vi "3D Point Cloud.vi"(0 "3D Information Cluster (X,Y,Z)":cluster{dbl[], dbl[], dbl[]}) -> ()   [LabVIEW 2010, in "Kinect_API.lvlib"]
doc: "This VI shows how to use the 3D Scatter Plot."
uses:
  Kinect_API.lvlib
  <vilib>/Math Plots/3D Math Plots/3D Scatter/3D Scatter XCtrl/3D Scatter.xctl
  <vilib>/Math Plots/3D Math Plots/3D Scatter/3D Scatter Datatype/Public/Plot Helper (Vector).vi
  <vilib>/Math Plots/3D Math Plots/3D Scatter/3D Scatter Datatype/3D Scatter Datatype.lvclass
panel:
  out "3D Scatter":refnum<class "3D Plot Datatype.lvclass">[](xcontrol)
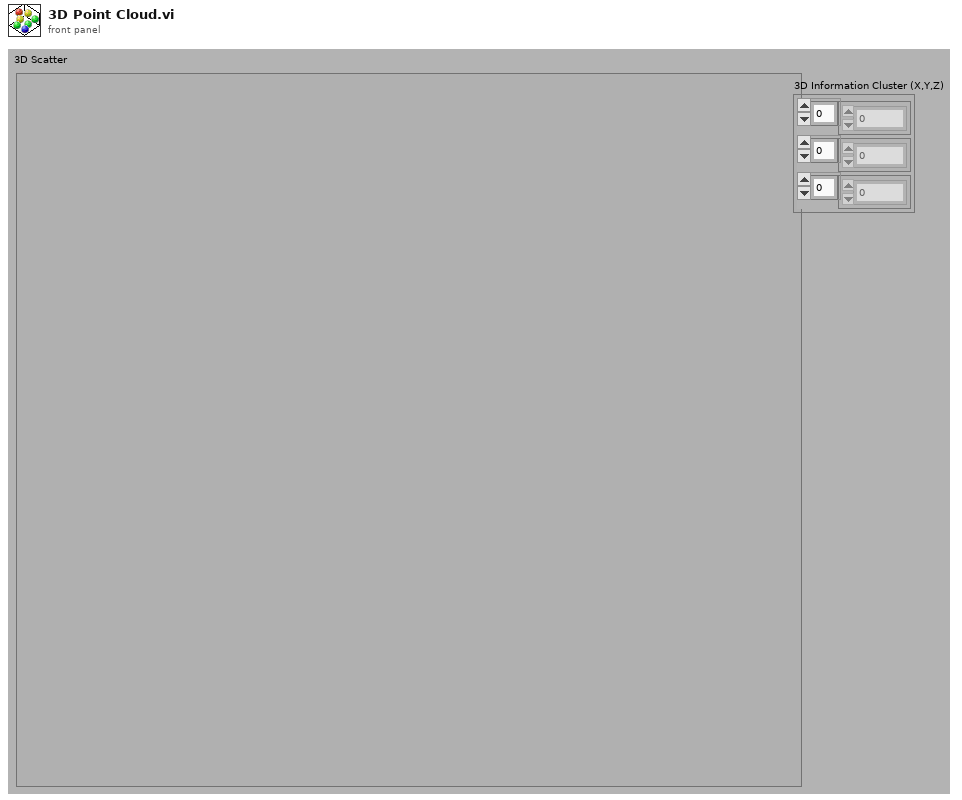
[diagram p1: front panel]
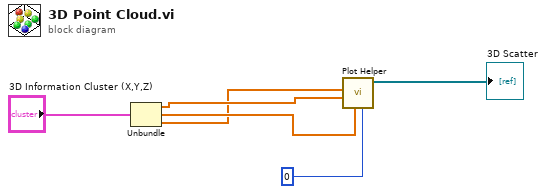
[diagram p0: block diagram]
diagram:
  n1 = Unbundle("3D Information Cluster (X,Y,Z)") -> (w2:dbl[], w3:dbl[], w1:dbl[])
  n2 = call-poly <vilib>:"Plot Helper.vi"("Plot ID"=0, "z vector"=w3, "y vector"=w2, "x vector"=w1) -> ("3D Plot lvclass Array out"=→"3D Scatter":refnum<class "3D Plot Datatype.lvclass">[])  [unwired: 2 in, 5 out]
